vi "CCM-Read Connection Tables (I32, by device).vi"(0 "Path In":path, 5 "Channels By Device":cluster{"Out":string[], "In":string[]}[](array[cluster]), 7 "Channels (1D)":cluster{"Out":string[], "In":string[]}, 11 "error in (no error)":errorcluster, 12 "Endpoints":cluster{"Name":string[]}[](array[cluster])) -> (4 "Path Out":path, 6 "Tables By Device":T1(array[cluster]), 15 "error out":errorcluster)   [LabVIEW 2020]
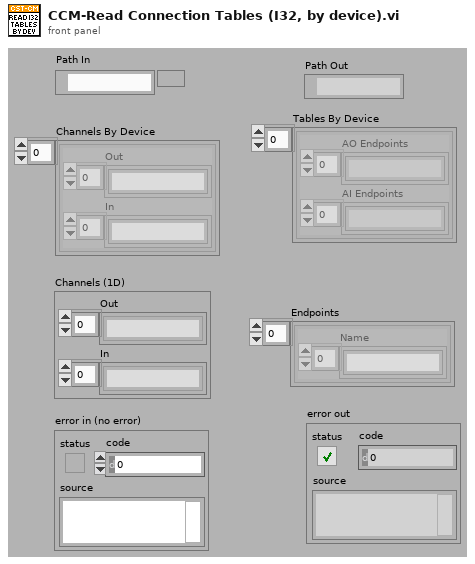
[diagram p1: front panel]
types:
  T1 = cluster{"AO Endpoints":string[], "AI Endpoints":string[]}[]
  T2 = cluster{"Endpoints (by channel)":string[], "Endpoints (by channel)":string[]}
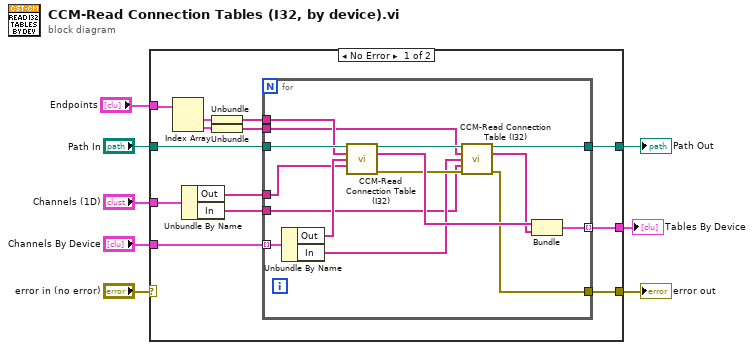
[diagram p0: block diagram]
diagram:
  n1 = case shown="No Error" "error in (no error)" {
    selector: "error in (no error)" -> [_ w38]
    tunnel: "Channels By Device" -> [w21 _]
    tunnel: "Path In" -> [w20 w37]
    tunnel: [w18 w38] -> w5
    tunnel: [w19 w37] -> w4
    tunnel: [w17 _] -> w3
    tunnel: "Channels (1D)" -> [w16 _]
    tunnel: "Endpoints" -> [w13 _]
    frame No Error {
      n2 = Index Array(array=w13) -> (element #1=w12:cluster{"Name":string[]}, element #2=w10:cluster{"Name":string[]})  [unwired: 2 in]
      n3 = Unbundle By Name(w16) -> ("Out"=w15:string[], "In"=w14:string[])
      n4 = Unbundle(w12) -> ("Name"=w11:string[])
      n5 = Unbundle(w10) -> ("Name"=w9:string[])
      n6 = for {
        tunnel: w21 -> [w36] mode=indexing
        tunnel: w20 -> [w34]
        tunnel: [w29] -> w19
        tunnel: [w32] -> w17 mode=indexing
        tunnel: [w27] -> w18
        tunnel: w15 -> [w25]
        tunnel: w14 -> [w24]
        tunnel: w11 -> [w23]
        tunnel: w9 -> [w22]
        n7 = Unbundle By Name(w36) -> ("Out"=w35:string[], "In"=w28:string[])
        n8 = call "CCM-Read Connection Table (I32).vi"("Path In"=w34, "Endpoints"=w23, "IOChannels"=w35, "Channel Names"=w25) -> ("Path Out"=w31:path, "Endpoints (by channel)"=w33:string[], "error out"=w30:errorcluster)  [unwired: 8 in, 1 out]
        n9 = call "CCM-Read Connection Table (I32).vi"("Path In"=w31, "Endpoints"=w22, "IOChannels"=w28, "Channel Names"=w24, "error in (no error)"=w30) -> ("Path Out"=w29:path, "Endpoints (by channel)"=w26:string[], "error out"=w27:errorcluster)  [unwired: 7 in, 1 out]
        n10 = Bundle("Endpoints (by channel)"=w33, "Endpoints (by channel)"=w26) -> (w32:T2)  [unwired: 1 in]
      }
    }
    frame Error {
    }
  }
  "error out" <- w5
  "Path Out" <- w4
  "Tables By Device" <- w3
